vi "test Multi FPGA Feature Toggle Removal.vi"(8 "error in (no error)":errorcluster, 11 "TestCase in":refnum<class "Mutation Test Case.lvclass">) -> (0 "error out":errorcluster, 3 "TestCase out":refnum<class "Mutation Test Case.lvclass">)   [LabVIEW 2019, in "Mutation Test Case.lvclass"]
uses:
  Mutation Test Case.lvclass
  Shared/Properties.vi
  <vilib>/NI VeriStand/Custom Device API/Get Item Property (Boolean).vi
  <vilib>/addons/_JKI Toolkits/VI Tester/TestCase.llb/TestCase.lvclass
  System Explorer/Engine Simulation Toolkit System Explorer.lvlib
  Shared/Engine Simulation Toolkit Shared.lvlib
  <vilib>/NI VeriStand/Custom Device API/Custom Device API.lvlib
  C:/Program Files (x86)/National Instruments/LabVIEW 2019/vi.lib/addons/_JKI Toolkits/VI Tester/TestCase.llb/TestCase.lvclass
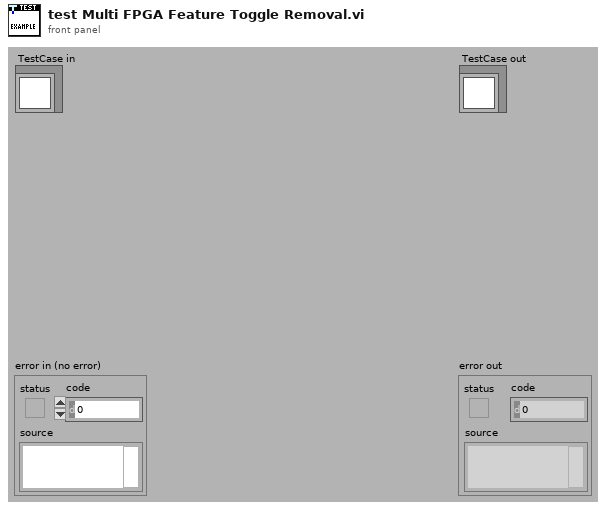
[diagram p1: front panel]
types:
  T1 = typedef "Custom Device API.lvlib/Custom Device Item Ref.ctl" = u64
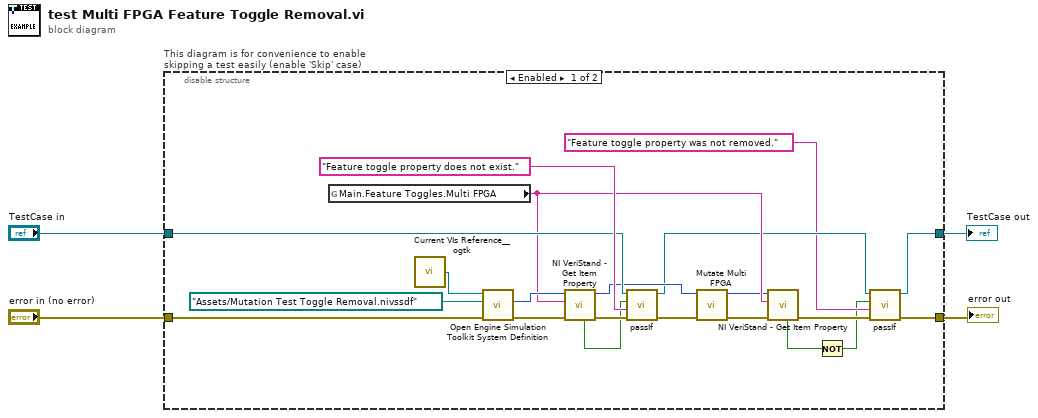
[diagram p0: block diagram]
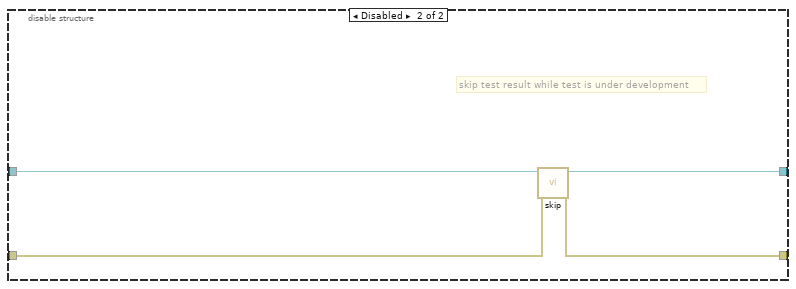
[diagram p2: hidden frame]
diagram:
  n1 = disable-structure "This diagram is for convenience to enable skipping a test easily (enable 'Skip' case)" shown="Enabled" {
    disable-tunnel: "TestCase in" -> [w16 w29]
    disable-tunnel: [w7 w27] -> w1
    disable-tunnel: [w9 w28] -> w3
    disable-tunnel: "error in (no error)" -> [w21 w26]
    frame Enabled {
      n2 = global read "Properties.vi" "Main.Feature Toggles.Multi FPGA"() -> (w14:string)
      n3 = call <userlib>:"Current VIs Reference__ogtk.vi"() -> ("Current VI's reference"=w25:refnum<vi>)  [unwired: 5 in]
      n4 = call "Open Engine Simulation Toolkit System Definition.vi"("error in (no error)"=w21, "System Definition Path"=path "Assets/Mutation Test Toggle Removal.nivssdf" ("Absolute or Relative Path"), "Current VI in"=w25) -> ("error out"=w20:errorcluster, "Engine Simulation Toolkit NodeID"=w19:u64)  [unwired: 6 in, 1 out]
      n5 = call-poly <vilib>:"NI VeriStand - Get Item Property.vi"("error in (no error)"=w20, "Property Name"=w14, "Item Ref in"=w19) -> ("error out"=w23:errorcluster, "Item Ref out"=w15:T1, "Found?"=w18:bool)  [unwired: 5 in, 1 out]
      n6 = call-dynamic "passIf.vi"("error in (no error)"=w23, "message (\"\")"="Feature toggle property does not exist." ("message (\"\")"), "pass"=w18, "TestCase in"=w16) -> ("error out"=w17:errorcluster, "TestCase out"=w8:refnum<class "Mutation Test Case.lvclass">)  [unwired: 6 in]
      n7 = call "Mutate Multi FPGA.vi"("error in (no error)"=w17, "Device Ref in"=w15) -> ("error out"=w12:errorcluster, "Device Ref out"=w13:T1)  [unwired: 8 in]
      n8 = call-poly <vilib>:"NI VeriStand - Get Item Property.vi"("error in (no error)"=w12, "Property Name"=w14, "Item Ref in"=w13) -> ("error out"=w10:errorcluster, "Found?"=w11:bool)  [unwired: 5 in, 2 out]
      n9 = Not(x=w11) -> (.not. x?=w5:bool)
      n10 = call-dynamic "passIf.vi"("error in (no error)"=w10, "message (\"\")"="Feature toggle property was not removed." ("message (\"\")"), "pass"=w5, "TestCase in"=w8) -> ("error out"=w9:errorcluster, "TestCase out"=w7:refnum<class "Mutation Test Case.lvclass">)  [unwired: 6 in]
    }
    frame Disabled {
      # "skip test result while test is under development"
      n11 = call <vilib>:"skip.vi"("error in (no error)"=w26, "TestCase in"=w29) -> ("error out"=w28:errorcluster, "TestCase out"=w27:refnum<class "Mutation Test Case.lvclass">)  [unwired: 8 in]
    }
  }
  "error out" <- w3
  "TestCase out" <- w1
